vi "ChildImplementationINIKey--Constant.vi"() -> (3 "ChildImplementationPathKey":string)   [LabVIEW 2021, in "IconEditorDefaultPlugin.lvlib" / "IconEditorDefaultPlugin.lvclass"]
uses:
  <resource>/plugins/NIIconEditor/UI/Default/IconEditorDefaultPlugin.lvclass
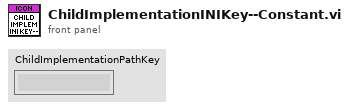
[diagram p1: front panel]
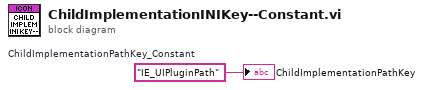
[diagram p0: block diagram]
diagram:
  w1 = "IE_UIPluginPath"  # ChildImplementationPathKey_Constant
  "ChildImplementationPathKey" <- w1
